vi "SortableDateTimes.vi"(11 "seconds since 1Jan1904":timestamp) -> (1 "dateTime":T1(array[cluster]), 3 "spreadsheetDateTimes":string)   [LabVIEW 2020]
uses:
  <vilib>/Utility/miscctls.llb/LVDateTimeRec.ctl
panel:
  out "DayOfYear":string
  out "sortableDate":string
  out "SecondsSinceMidnight":dbl
  out "DayOfMonth":string
  out "Month":string
  out "DayOfWeek":string
  out "DayName":string
  out "Year":string
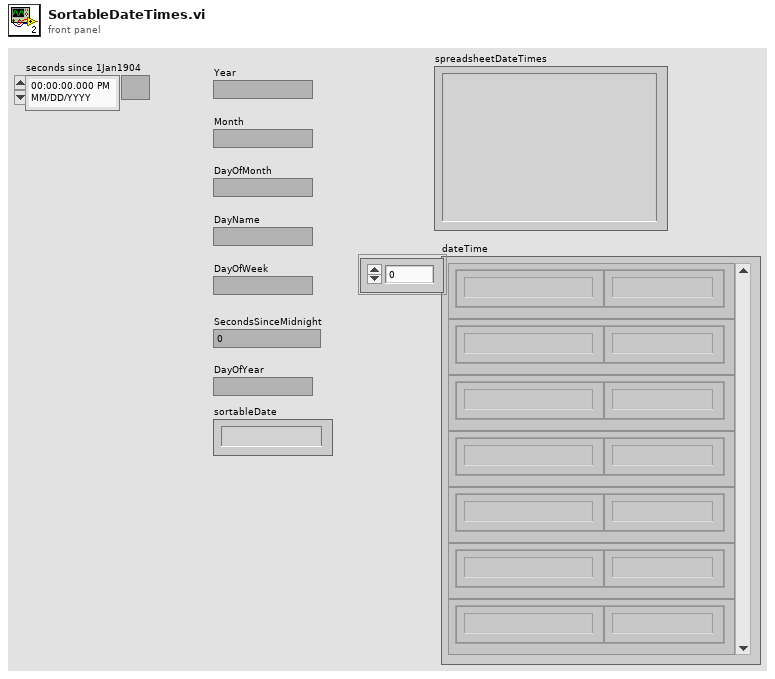
[diagram p1: front panel]
types:
  T1 = cluster{"Label.Text":string, "date/time string":string}[]
  T2 = typedef "LVDateTimeRec.ctl" = cluster{"fractional second":dbl, "second":i32, "minute":i32, "hour":i32, "day of month":i32, "month":i32, "year":i32, "day of week":i32, "day of year":i32, "DST":i32}
  T3 = cluster{"Label.Text":string, "date/time string":string}
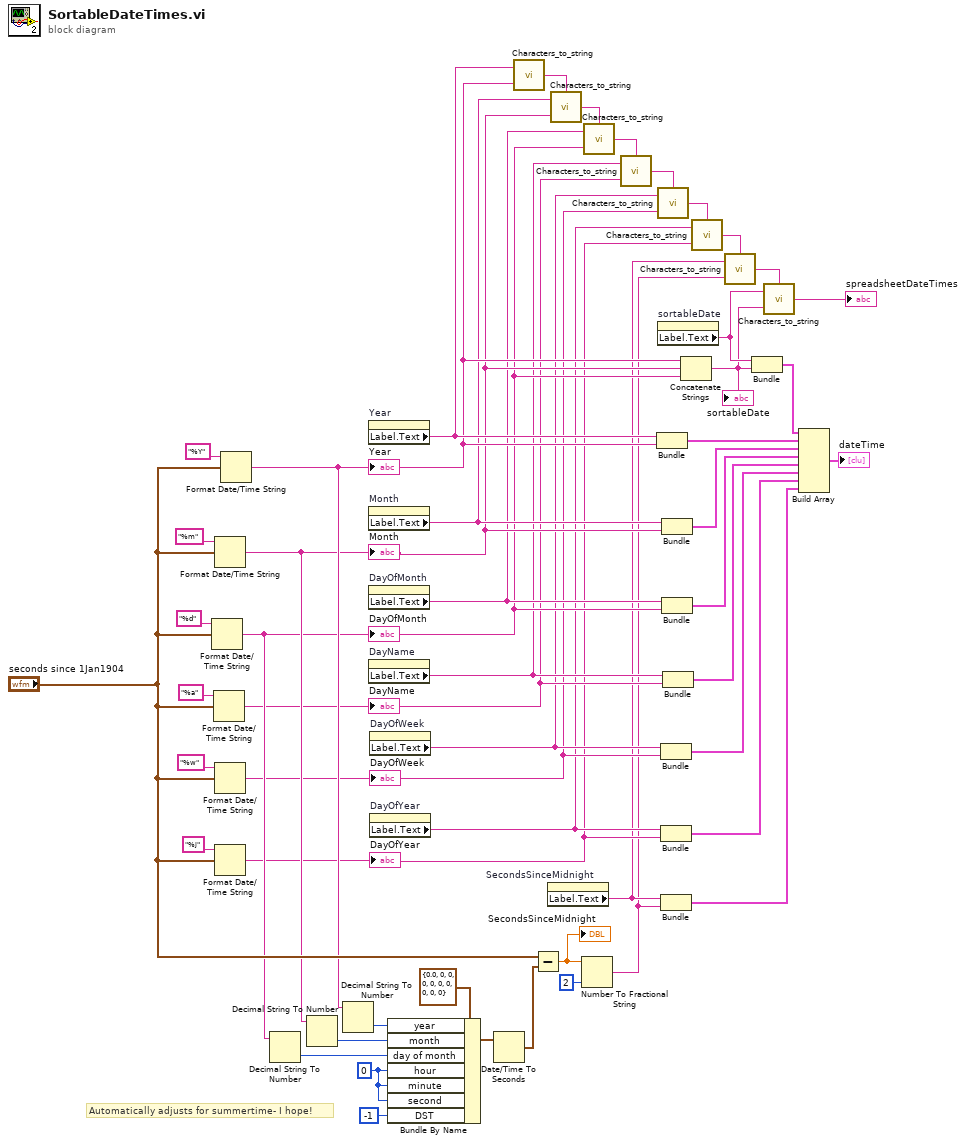
[diagram p0: block diagram]
diagram:
  w49 = 0 ("hour")
  # "Automatically adjusts for summertime- I hope!"
  n1 = Format Date/Time String(time format string (%c)="%d", seconds (now)="seconds since 1Jan1904") -> (date/time string=w12:string)  [unwired: 1 in]
  "DayOfMonth" <- w12
  n2 = Format Date/Time String(time format string (%c)="%a", seconds (now)="seconds since 1Jan1904") -> (date/time string=w10:string)  [unwired: 1 in]
  "DayName" <- w10
  n3 = Format Date/Time String(time format string (%c)="%m", seconds (now)="seconds since 1Jan1904") -> (date/time string=w14:string)  [unwired: 1 in]
  "Month" <- w14
  n4 = Format Date/Time String(time format string (%c)="%w", seconds (now)="seconds since 1Jan1904") -> (date/time string=w8:string)  [unwired: 1 in]
  "DayOfWeek" <- w8
  n5 = Format Date/Time String(time format string (%c)="%j", seconds (now)="seconds since 1Jan1904") -> (date/time string=w6:string)  [unwired: 1 in]
  "DayOfYear" <- w6
  n6 = Format Date/Time String(time format string (%c)="%Y", seconds (now)="seconds since 1Jan1904") -> (date/time string=w23:string)  [unwired: 1 in]
  "Year" <- w23
  n7 = Decimal String To Number(string=w12) -> (number=w47:i32)  [unwired: 2 in, 1 out]
  n8 = Decimal String To Number(string=w14) -> (number=w46:i32)  [unwired: 2 in, 1 out]
  n9 = Decimal String To Number(string=w23) -> (number=w45:i32)  [unwired: 2 in, 1 out]
  n10 = property on="Year" class="Str"() -> ("Label.Text"=w24:string)  [unwired: 2 in, 2 out]
  n11 = property on="Month" class="Str"() -> ("Label.Text"=w15:string)  [unwired: 2 in, 2 out]
  n12 = property on="DayOfMonth" class="Str"() -> ("Label.Text"=w13:string)  [unwired: 2 in, 2 out]
  n13 = property on="DayName" class="Str"() -> ("Label.Text"=w11:string)  [unwired: 2 in, 2 out]
  n14 = property on="DayOfWeek" class="Str"() -> ("Label.Text"=w9:string)  [unwired: 2 in, 2 out]
  n15 = property on="DayOfYear" class="Str"() -> ("Label.Text"=w7:string)  [unwired: 2 in, 2 out]
  n16 = Bundle By Name(cluster=T2 {"fractional second"=0.0, "second"=0, "minute"=0, "hour"=0, "day of month"=0, "month"=0, "year"=0, "day of week"=0, "day of year"=0, "DST"=0} ("date time rec"), "year"=w45, "month"=w46, "day of month"=w47, "hour"=w49, "minute"=w49, "second"=w49, "DST"=-1) -> (w43:T2)
  n17 = Date/Time To Seconds(2:w43) -> (0:w48:timestamp)  [unwired: 1 in]
  n18 = call "Characters_to_string.vi"("Characters to write"=w23, "Label for characters"=w24) -> ("Output string"=w22:string)  [unwired: 1 in]
  n19 = Subtract(x="seconds since 1Jan1904", y=w48) -> (x-y=w37:dbl)
  "SecondsSinceMidnight" <- w37
  n20 = property on="SecondsSinceMidnight" class="DigNum (strict)"() -> ("Label.Text"=w5:string)  [unwired: 2 in, 2 out]
  n21 = call "Characters_to_string.vi"("stringIn"=w22, "Characters to write"=w14, "Label for characters"=w15) -> ("Output string"=w21:string)
  n22 = Number To Fractional String(number=w37, precision (6)=i16 2) -> (F-format string=w4:string)  [unwired: 2 in]
  n23 = call "Characters_to_string.vi"("stringIn"=w21, "Characters to write"=w12, "Label for characters"=w13) -> ("Output string"=w20:string)
  n24 = call "Characters_to_string.vi"("stringIn"=w20, "Characters to write"=w10, "Label for characters"=w11) -> ("Output string"=w19:string)
  n25 = Bundle("Label.Text"=w24, "date/time string"=w23) -> (w35:T3)  [unwired: 1 in]
  n26 = call "Characters_to_string.vi"("stringIn"=w19, "Characters to write"=w8, "Label for characters"=w9) -> ("Output string"=w18:string)
  n27 = property on="sortableDate" class="Str"() -> ("Label.Text"=w3:string)  [unwired: 2 in, 2 out]
  n28 = Bundle("Label.Text"=w9, "date/time string"=w8) -> (w31:T3)  [unwired: 1 in]
  n29 = Bundle("Label.Text"=w7, "date/time string"=w6) -> (w25:T3)  [unwired: 1 in]
  n30 = Bundle("Label.Text"=w5, w4) -> (w26:cluster{"Label.Text":string, string})  [unwired: 1 in]
  n31 = Bundle("Label.Text"=w15, "date/time string"=w14) -> (w34:T3)  [unwired: 1 in]
  n32 = Bundle("Label.Text"=w13, "date/time string"=w12) -> (w33:T3)  [unwired: 1 in]
  n33 = Bundle("Label.Text"=w11, "date/time string"=w10) -> (w32:T3)  [unwired: 1 in]
  n34 = Concatenate Strings(w23, w14, w12) -> (w2:string)
  "sortableDate" <- w2
  n35 = call "Characters_to_string.vi"("stringIn"=w18, "Characters to write"=w6, "Label for characters"=w7) -> ("Output string"=w17:string)
  n36 = call "Characters_to_string.vi"("stringIn"=w17, "Characters to write"=w4, "Label for characters"=w5) -> ("Output string"=w16:string)
  n37 = Bundle("Label.Text"=w3, w2) -> (w29:cluster{"Label.Text":string, string})  [unwired: 1 in]
  n38 = call "Characters_to_string.vi"("stringIn"=w16, "Characters to write"=w2, "Label for characters"=w3) -> ("Output string"=→"spreadsheetDateTimes":string)
  n39 = Build Array(w29, w35, w34, w33, w32, w31, w25, w26) -> (→"dateTime":T1)
